vi "VisualizeAppLSE.vi"() -> ()   [LabVIEW 2014, in "Visualization.lvlib" / "VisualizeAppLSE.lvclass"]
uses:
  VisualizeAppLSE.lvclass
  Modules/AppModule/PublicAPI/Arguments/Broadcasts/clStatUpdate.ctl
  VisializeBase_class/Requests/clUserEventType.ctl
  Modules/EventPlugins/EventPluginBaseClass/TypeDefs/clEvtReportArray.ctl
  Modules/EventPlugins/EventPluginBaseClass/TypeDefs/clEvtReport.ctl
  VisualizeAppBase_class.lvclass/VisualizeAppBase_class.ctl
  Modules/AppPlugins/LSEPlugin/PublicAPI/Typedefs/LSEOutput.ctl
  Modules/AppPlugins/LSEPlugin/PublicAPI/Typedefs/LSEConfig.ctl
  VisualizeAppLSE.lvclass/VisualizeAppLSE.ctl
  <vilib>/event_ctls.llb/usereventprio.ctl
  VisualizeAppBase/Accessors/Write clEvtReportArray.vi
  Accessors/Write LSEOutput.vi
  Accessors/Read LSEOutput.vi
  Accessors/Write tve.vi
  Accessors/Write EvtParams.vi
  VisualizeAppBase/Accessors/Read clEvtReportArray.vi
  Accessors/Read tve.vi
  <vilib>/Analysis/BLAS.llb/dnrm2 - Vector 2-Norm (DBL).vi
  <vilib>/Utility/error.llb/Error Cluster From Error Code.vi
  <vilib>/ErrorRing/Error Ring.xnode
  <userlib>/NIST/NISTErrorLib/NISTErrorLib.lvlib
  VisializeBase_class/VisualizeBase_class.lvclass
  Modules/AppModule/AppModule.lvlib
  Modules/EventPlugins/EventPluginBaseClass/EventPluginBaseClass.lvclass
  Modules/PmuImpairModule/PmuImpairModule.lvlib
  Modules/EventModule/EventModule.lvlib
  <vilib>/Analysis/NI_AALBLAS.lvlib
  Modules/AppPlugins/LSEPlugin/LSEPlugin.lvclass
panel:
  out "TVE":waveform(dbl)(graph)
  out "PMU Number":dbl
  in  "Bus Number":u16(ring) items=["1"=1, "2"=2, "3"=3, "4"=4, "5"=5]
  out "IEEE Bus System":u32
  out "% Observed Buses":dbl
  out "Angle estimate":waveform(dbl)[](graph)
  out "Magnitude estimate":waveform(dbl)[](graph)
  out "Event Parameters":dbl[][](array[numeric])
  in  "btnStop":bool
  out "Status Broadcasts":string
  in  "QueName":string="VisAppQue"
  out "TSE":waveform(dbl)[](graph)
  in  "restart VI":bool
  out "Error Array":errorcluster[][](array[cluster])
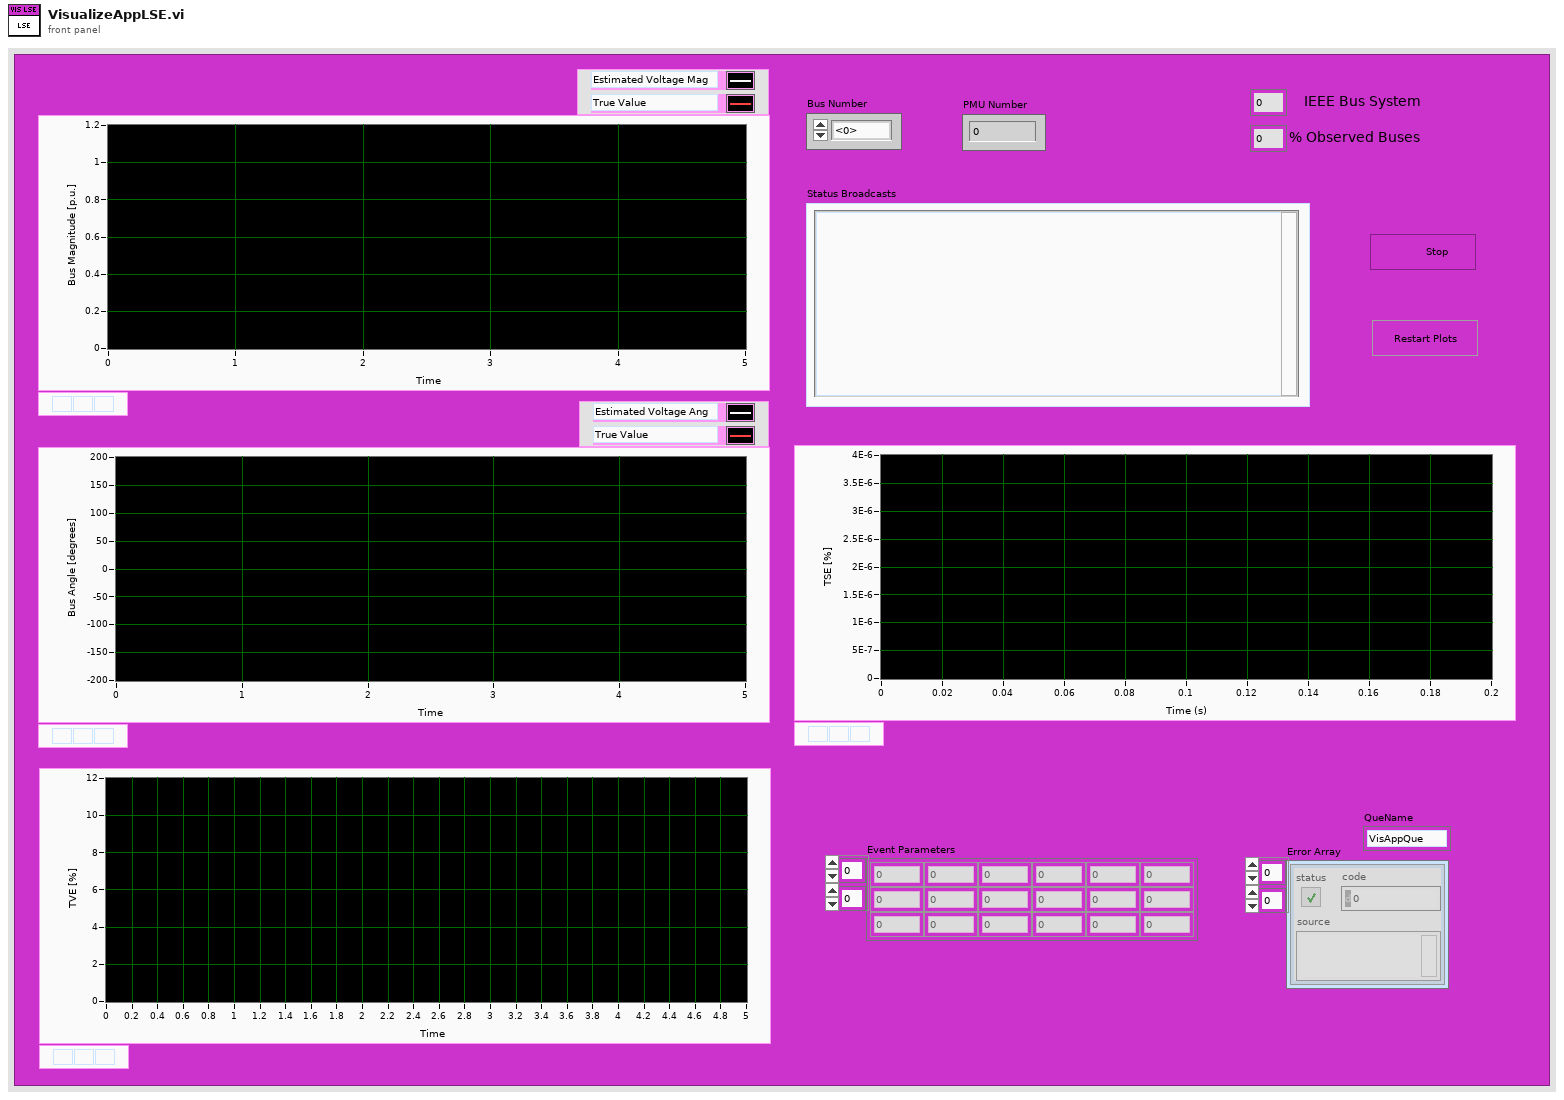
[diagram p1: front panel]
types:
  T1 = typedef "EventPlugins.lvlib/EventPluginBaseClass.lvclass/clEvtReportArray.ctl" = T2[]
  T2 = typedef "EventPlugins.lvlib/EventPluginBaseClass.lvclass/clEvtReport.ctl" = cluster{"Timestamp":dbl, "Synx":cdb[], "Freq":dbl, "ROCOF":dbl, "ID":i16}
  T3 = typedef "AppPlugins.lvlib/LSEPlugin.lvclass/LSEOutput.ctl" = cluster{"SystemVoltagesRef":cdb[][], "Vestimate":cdb[][], "LSEConfig":T4, "Bus":dbl[]}
  T4 = typedef "AppPlugins.lvlib/LSEPlugin.lvclass/LSEConfig.ctl" = cluster{"NoiseVariance":dbl, "IEEESystem":u32, "PMULocations":u32[], "Vindex":i32, "Iindex":i32, "DynamicRef":string}
  T5 = typedef "Visualization.lvlib/VisualizeBase_class.lvclass/clUserEventType.ctl" = cluster{"BusIndex":i8, "Data":variant}
  T6 = typedef "usereventprio.ctl" = enum32{"high priority", "normal priority"}
  T7 = typedef "AppModule.lvlib/clStatUpdate.ctl" = cluster{"Status":string}
  T8 = typedef "Visualization.lvlib/VisualizeBase_class.lvclass/clRequestEvents.ctl" = cluster{"StopRequest":refnum<user-event>}
  T9 = typedef "AppModule.lvlib/clBroadcastEvents.ctl" = cluster{"DidInit":refnum<user-event>, "StatusUpdate":refnum<user-event>, "ErrorReport":refnum<user-event>, "DidStop":refnum<user-event>, "PathToINI":refnum<user-event>, "InputData":refnum<user-event>, "OutputData":refnum<user-event>, "BcAppInfo":refnum<user-event>, "ConfigData":refnum<user-event>}
  T10 = typedef "PmuImpairModule.lvlib/clBroadcastEvents.ctl" = cluster{"DidInit":refnum<user-event>, "StatusUpdate":refnum<user-event>, "ErrorReport":refnum<user-event>, "DidStop":refnum<user-event>, "ImpairConfig":refnum<user-event>, "ImpairParams":refnum<user-event>, "ImpairReports":refnum<user-event>, "PathToPlugin":refnum<user-event>, "BusNumber":refnum<user-event>}
  T11 = typedef "EventModule.lvlib/clBroadcastEvents.ctl" = cluster{"DidInit":refnum<user-event>, "StatusUpdate":refnum<user-event>, "ErrorReport":refnum<user-event>, "DidStop":refnum<user-event>, "ReadEvtConfig":refnum<user-event>, "ReadTimeArray":refnum<user-event>, "ReadEvtParams":refnum<user-event>, "GetEvtReportArray":refnum<user-event>, "ReadPathToPlugin":refnum<user-event>, "GetEvtSignal":refnum<user-event>, "ReadBusNumber":refnum<user-event>}
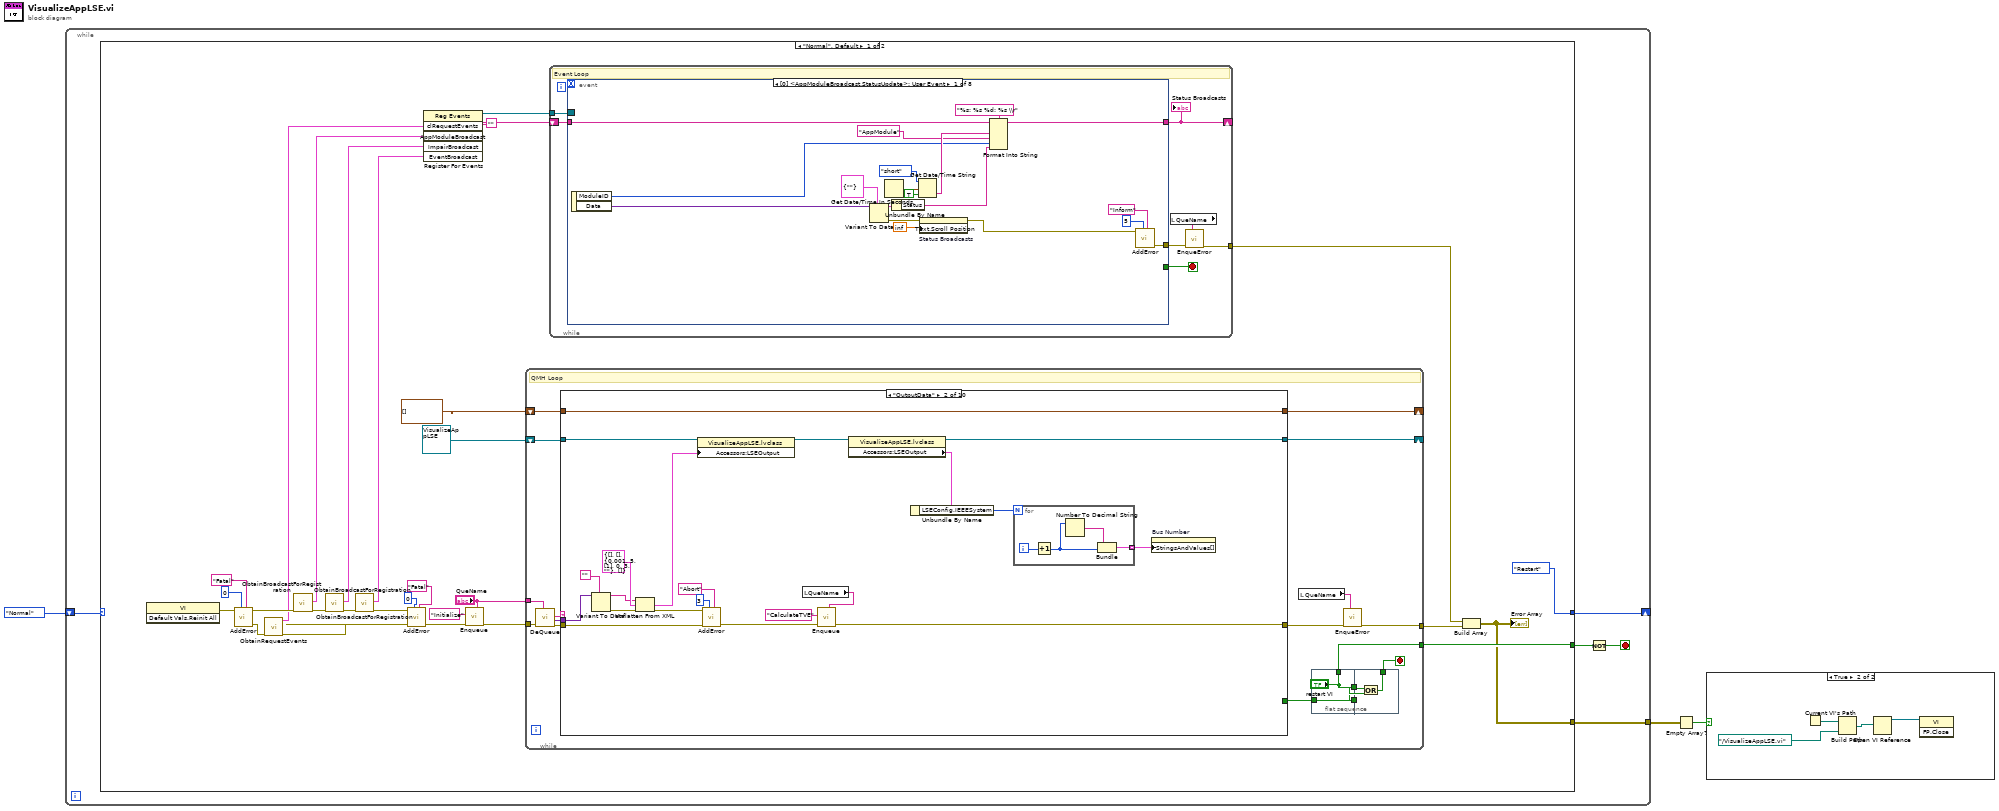
[diagram p0: block diagram]
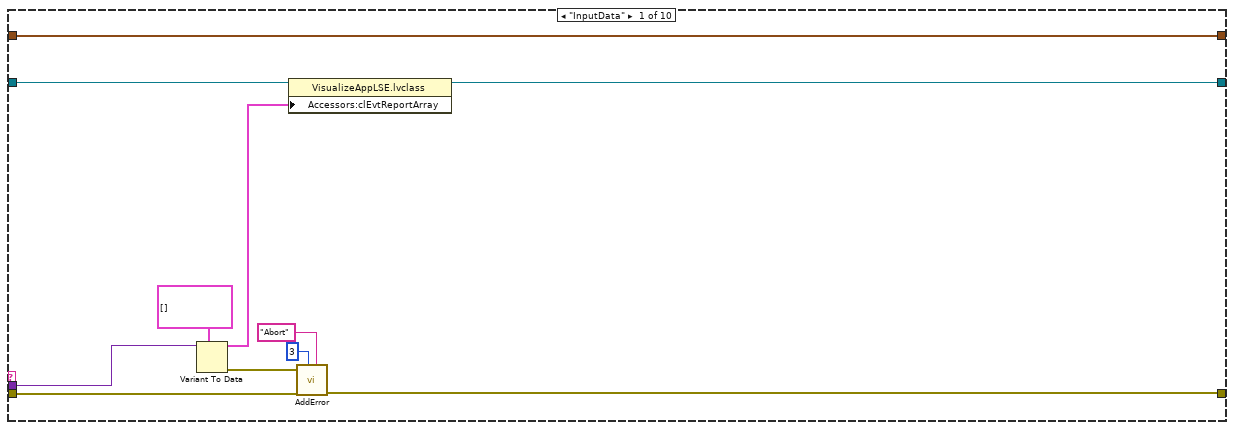
[diagram p3: hidden frame]
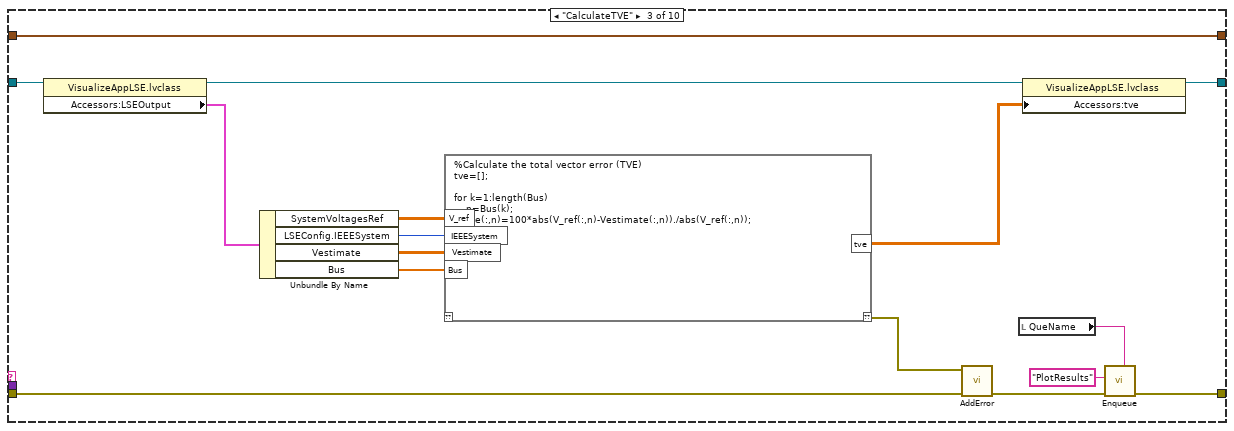
[diagram p4: hidden frame]
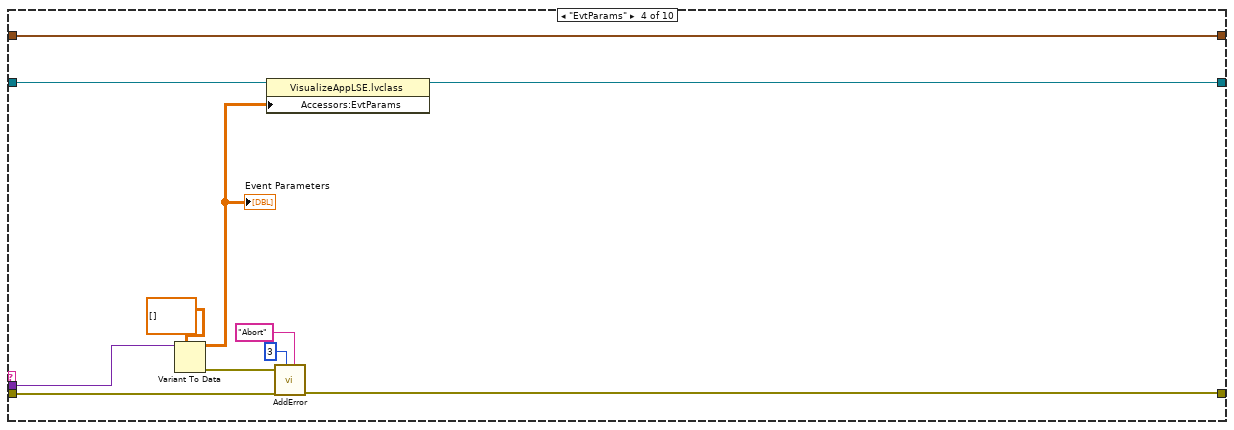
[diagram p5: hidden frame]
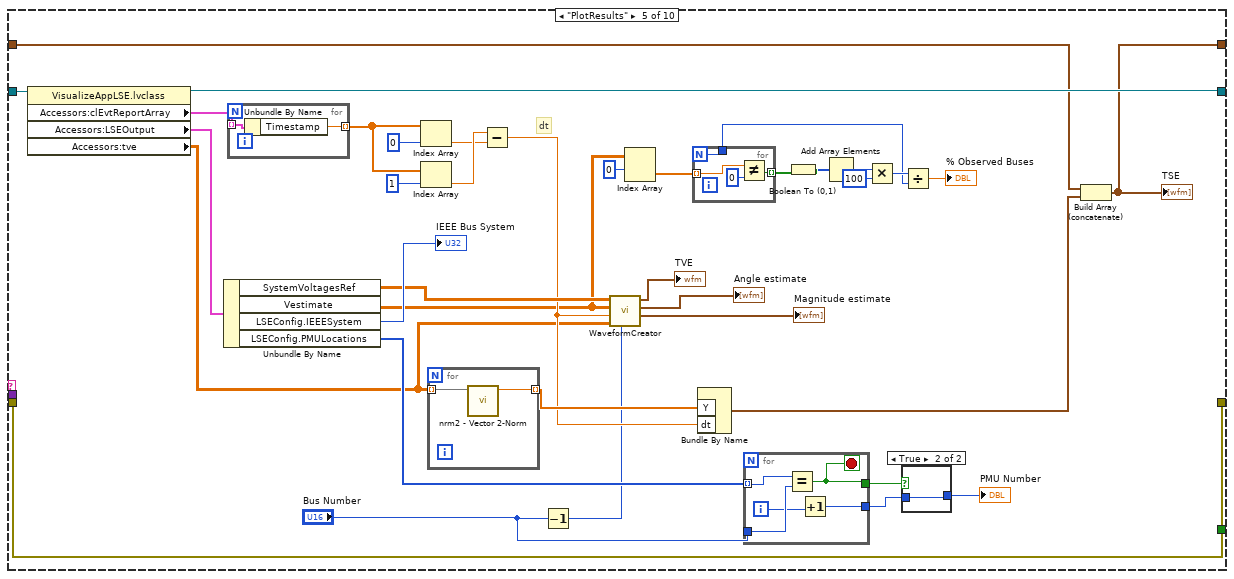
[diagram p6: hidden frame]
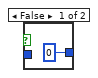
[diagram p7: hidden frame]
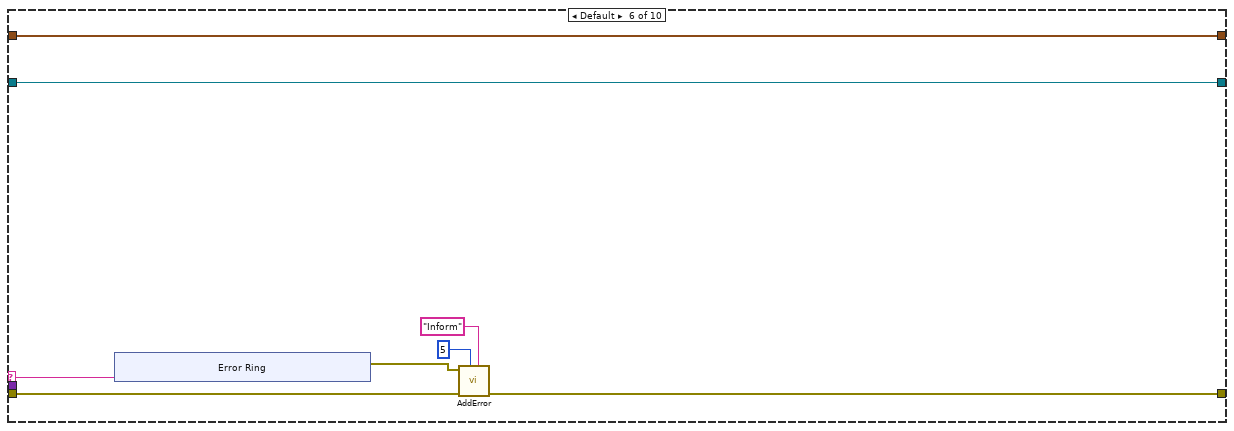
[diagram p8: hidden frame]
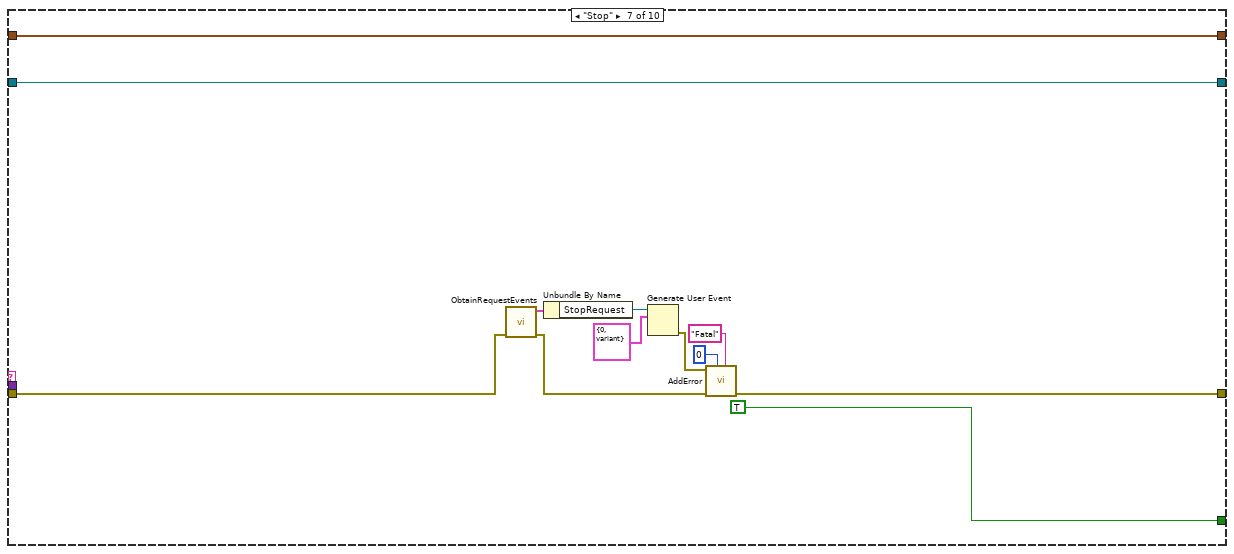
[diagram p9: hidden frame]
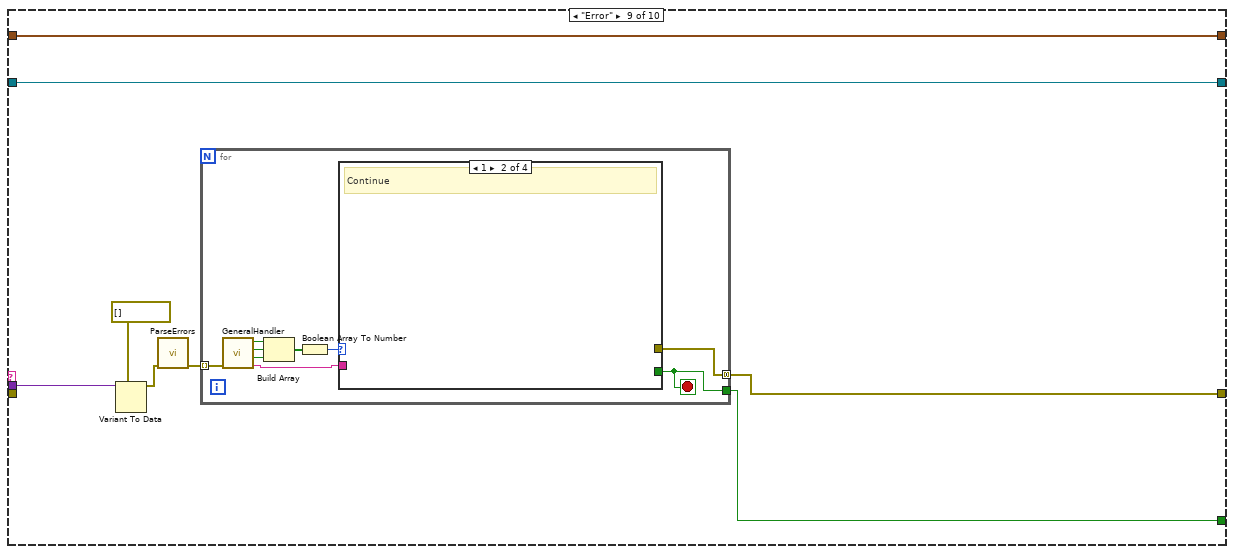
[diagram p11: hidden frame]
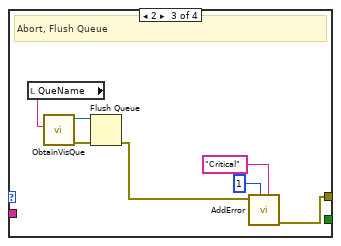
[diagram p13: hidden frame]
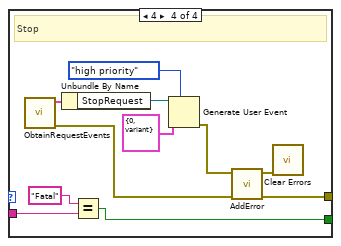
[diagram p14: hidden frame]
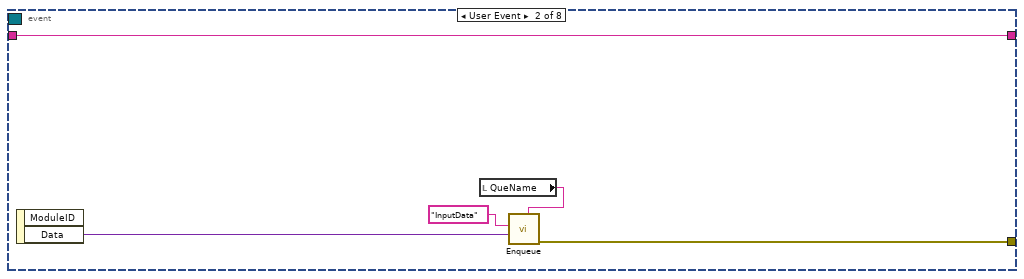
[diagram p16: hidden frame]
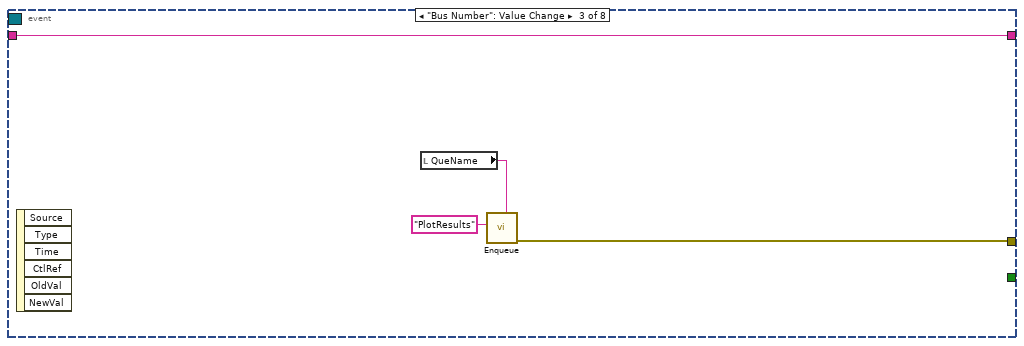
[diagram p17: hidden frame]
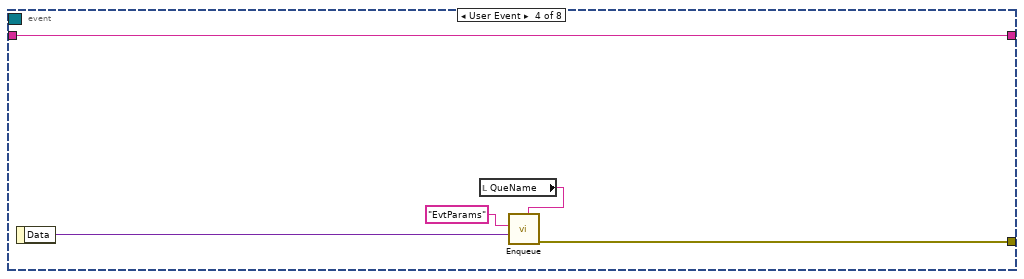
[diagram p18: hidden frame]
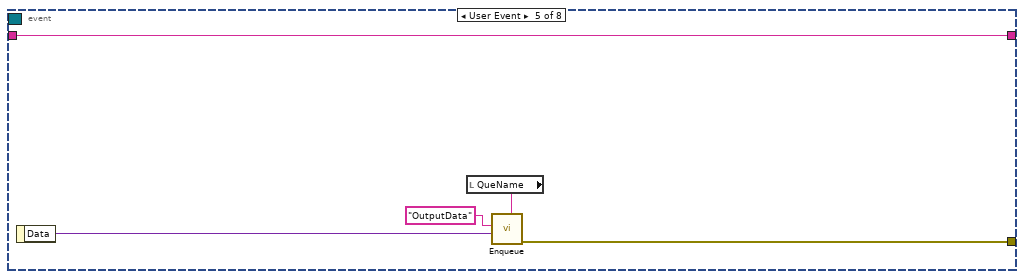
[diagram p19: hidden frame]
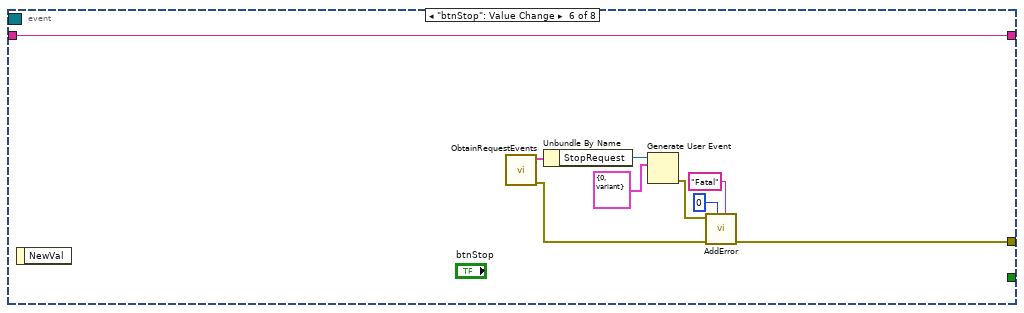
[diagram p20: hidden frame]
diagram:
  n1 = while {
    shift-right: [w5] -> _
    shift-left: enum16{"Normal", "Restart"}."Normal" -> [w6]
    tunnel: [w4] -> w1
    stop <- w7 stop-if-true
    n2 = case shown="\"Normal\", Default" w6 {
      tunnel: [w13 TRUE] -> w8
      tunnel: [enum16{"Normal", "Restart"}."Restart" enum16{"Normal", "Restart"}."Normal"] -> w5
      tunnel: [w10 errorcluster[][] []] -> w4
      frame "Normal", Default {
        n3 = invoke class="VI" method="Default Vals.Reinit All"() -> (error out=w19:errorcluster)  [unwired: 3 in, 2 out]
        n4 = call <userlib>:"AddError.vi"("Severity"="Fatal", "Priority"=u8 0, "error in (no error)"=w19) -> ("ErrorArray"=w34:errorcluster[], "error out"=w33:errorcluster)  [unwired: 7 in]
        n5 = call "ObtainRequestEvents.vi"("Error"=w34) -> ("Error"=w30:errorcluster[], "clRequestEvents"=w32:T8)  [unwired: 9 in]
        n6 = call "ObtainBroadcastForRegistration.vi"("error in (no error)"=w33) -> ("error out"=w18:errorcluster, "AppModuleBroadcast"=w31:T9)  [unwired: 9 in]
        n7 = call "ObtainBroadcastForRegistration.vi"("error in (no error)"=w18) -> ("error out"=w17:errorcluster, "ImpairBroadcast"=w16:T10)  [unwired: 9 in]
        n8 = call "ObtainBroadcastForRegistration.vi"("error in (no error)"=w17) -> ("error out"=w15:errorcluster, "EventBroadcast"=w14:T11)  [unwired: 9 in]
        n9 = call <userlib>:"AddError.vi"("Severity"="Fatal", "Priority"=u8 0, "ErrorArray"=w30, "error in (no error)"=w15) -> ("ErrorArray"=w28:errorcluster[])  [unwired: 6 in, 1 out]
        n10 = register-events(w32, w31, w16, w14) -> (reference out=w23:refnum<event-registration>)  [unwired: 2 in, 1 out]
        n11 = call "Enqueue.vi"("QueName"="QueName", "Error"=w28, "Message"="Initialize") -> ("Error"=w25:errorcluster[])  [unwired: 8 in]
        n12 = while {
          tunnel: w25 -> [w53]
          tunnel: "QueName" -> [w52]
          tunnel: [w46] -> w22
          shift-right: [w44] -> _
          shift-left: refnum<class "VisualizeAppLSE.lvclass"> refnum ("Visualization.lvlib:VisualizeAppLSE.lvclass") -> [w45]
          shift-right: [w42] -> _
          shift-left: waveform(dbl)[] [] -> [w43]
          tunnel: [w41] -> w13
          stop <- w37 stop-if-true
          # "QMH Loop"
          n13 = call "DeQueue.vi"("QueName"=w52, "Error"=w53) -> ("Error"=w49:errorcluster[], "Data"=w50:variant, "Message"=w51:string)  [unwired: 7 in]
          n14 = case shown="\"OutputData\"" w51 {
            selector: w51 -> [_ _ _ _ _ w181 _ _ _ _]
            tunnel: w50 -> [w67 w89 _ w119 _ _ _ _ w208 _]
            tunnel: w49 -> [w63 w88 w99 w116 w124 w180 w192 w203 _ w239]
            tunnel: [w62 w84 w108 w115 w124 w176 w193 w203 w210 w239] -> w48
            tunnel: [_ _ _ _ _ _ TRUE _ w211 _] -> w39
            tunnel: w45 -> [w69 w90 w106 w121 w158 w175 w190 w202 w205 w240]
            tunnel: [w68 w79 w104 w120 w157 w175 w190 w202 w205 w240] -> w44
            tunnel: w43 -> [w59 w81 w107 w111 w155 w174 w189 w201 w204 w241]
            tunnel: [w59 w81 w107 w111 w146 w174 w189 w201 w204 w241] -> w42
            frame "InputData" {
              n15 = Variant To Data(type=T1 [] ("clEvtReportArray"), Variant=w67) -> (data=w65:T1, error out=w64:errorcluster)  [unwired: 1 in]
              n16 = property class="VisualizeAppLSE.lvclass"(reference=w69, "Accessors:clEvtReportArray"=w65) -> (reference out=w68:refnum<class "VisualizeAppLSE.lvclass">)  [unwired: 1 in, 1 out]
              n17 = call <userlib>:"AddError.vi"("Severity"="Abort", "Priority"=u8 3, "ErrorArray"=w63, "error in (no error)"=w64) -> ("ErrorArray"=w62:errorcluster[])  [unwired: 6 in, 1 out]
            }
            frame "OutputData" {
              n18 = Variant To Data(type="", Variant=w89) -> (data=w73:string, error out=w72:errorcluster)  [unwired: 1 in]
              n19 = Unflatten From XML(xml string=w73, type=T3 {"SystemVoltagesRef"=[], "Vestimate"=[], "LSEConfig"={"NoiseVariance"=0.001, "IEEESystem"=5, "PMULocations"=[1], "Vindex"=0, "Iindex"=3, "DynamicRef"=""}, "Bus"=[]} ("LSEOutput"), error in (no error)=w72) -> (value=w70:T3, error out=w71:errorcluster)
              n20 = property class="VisualizeAppLSE.lvclass"(reference=w90, "Accessors:LSEOutput"=w70) -> (reference out=w80:refnum<class "VisualizeAppLSE.lvclass">)  [unwired: 1 in, 1 out]
              n21 = call <userlib>:"AddError.vi"("Severity"="Abort", "Priority"=u8 3, "ErrorArray"=w88, "error in (no error)"=w71) -> ("ErrorArray"=w85:errorcluster[])  [unwired: 6 in, 1 out]
              n22 = local read "QueName"() -> (w82:string)
              n23 = call "Enqueue.vi"("QueName"=w82, "Error"=w85, "Message"="CalculateTVE") -> ("Error"=w84:errorcluster[])  [unwired: 8 in]
              n24 = property class="VisualizeAppLSE.lvclass"(reference=w80) -> (reference out=w79:refnum<class "VisualizeAppLSE.lvclass">, "Accessors:LSEOutput"=w78:T3)  [unwired: 1 in, 1 out]
              n25 = Unbundle By Name(w78) -> ("LSEConfig.IEEESystem"=w77:u32)
              n26 = for {
                N: w77 -> [_]
                tunnel: [w93] -> w76 mode=indexing
                i -> [w92]
                n27 = Increment(x=w92) -> (x+1=w91:i32)
                n28 = Number To Decimal String(number=w91) -> (decimal integer string=w94:string)  [unwired: 1 in]
                n29 = Bundle(w94, w91) -> (w93:cluster{string, i32})  [unwired: 1 in]
              }
              n30 = property on="Bus Number" class="Ring (strict)"("StringsAndValues[]"=w76) -> ()  [unwired: 2 in, 2 out]
            }
            frame "CalculateTVE" {
              n31 = property class="VisualizeAppLSE.lvclass"(reference=w106) -> (reference out=w105:refnum<class "VisualizeAppLSE.lvclass">, "Accessors:LSEOutput"=w97:T3)  [unwired: 1 in, 1 out]
              n32 = Unbundle By Name(w97) -> ("SystemVoltagesRef"=w95:cdb[][], "LSEConfig.IEEESystem"=w103:u32, "Vestimate"=w102:cdb[][], "Bus"=w101:dbl[])
              n33 = script code="%Calculate the total vector error (TVE)\ntve=[];\n\nfor k=1:length(Bus)\n    n=Bus(k);\n    tve(:,n)=100*abs(V_ref(:,n)-Vestimate(:,n))./abs(V_ref(:,n));  \nend"("V_ref"=w95, "IEEESystem"=w103, "Vestimate"=w102, "Bus"=w101) -> ("??"=w100:errorcluster, "tve"=w96:dbl[][])  [unwired: 1 in]
              n34 = call <userlib>:"AddError.vi"("ErrorArray"=w99, "error in (no error)"=w100) -> ("ErrorArray"=w98:errorcluster[])  [unwired: 8 in, 1 out]
              n35 = local read "QueName"() -> (w109:string)
              n36 = property class="VisualizeAppLSE.lvclass"(reference=w105, "Accessors:tve"=w96) -> (reference out=w104:refnum<class "VisualizeAppLSE.lvclass">)  [unwired: 1 in, 1 out]
              n37 = call "Enqueue.vi"("QueName"=w109, "Error"=w98, "Message"="PlotResults") -> ("Error"=w108:errorcluster[])  [unwired: 8 in]
            }
            frame "EvtParams" {
              n38 = Variant To Data(type=dbl[][] [], Variant=w119) -> (data=w118:dbl[][], error out=w117:errorcluster)  [unwired: 1 in]
              "Event Parameters" <- w118
              n39 = property class="VisualizeAppLSE.lvclass"(reference=w121, "Accessors:EvtParams"=w118) -> (reference out=w120:refnum<class "VisualizeAppLSE.lvclass">)  [unwired: 1 in, 1 out]
              n40 = call <userlib>:"AddError.vi"("Severity"="Abort", "Priority"=u8 3, "ErrorArray"=w116, "error in (no error)"=w117) -> ("ErrorArray"=w115:errorcluster[])  [unwired: 6 in, 1 out]
            }
            frame "PlotResults" {
              # "dt"
              n41 = property class="VisualizeAppLSE.lvclass"(reference=w158) -> (reference out=w157:refnum<class "VisualizeAppLSE.lvclass">, "Accessors:clEvtReportArray"=w153:T1, "Accessors:LSEOutput"=w152:T3, "Accessors:tve"=w122:dbl[][])  [unwired: 1 in, 1 out]
              n42 = Unbundle By Name(w152) -> ("SystemVoltagesRef"=w131:cdb[][], "Vestimate"=w128:cdb[][], "LSEConfig.IEEESystem"=→"IEEE Bus System":u32, "LSEConfig.PMULocations"=w127:u32[])
              n43 = for {
                tunnel: w153 -> [w173] mode=indexing
                tunnel: [w172] -> w149 mode=indexing
                n44 = Unbundle By Name(w173) -> ("Timestamp"=w172:dbl)
              }
              n45 = Index Array(array=w149, index=0) -> (element=w147:dbl)
              n46 = Index Array(array=w149, index=1) -> (element=w148:dbl)
              n47 = for {
                tunnel: [w170] -> w151 mode=indexing
                tunnel: w122 -> [w171] mode=indexing
                n48 = call-poly <vilib>:"nrm2 - Vector 2-Norm.vi"("x"=w171) -> ("dnrm2"=w170:dbl)  [unwired: 9 in, 1 out]
              }
              n49 = Subtract(x=w148, y=w147) -> (x-y=w130:dbl)
              n50 = Decrement(x="Bus Number") -> (x-1=w123:u16)
              n51 = call "WaveformCreator.vi"("BusNumber"=w123, "error"=w122, "dt"=w130, "Vestimate"=w128, "SystemVoltagesRef"=w131) -> ("MagnitudeEstimate"=→"Magnitude estimate":waveform(dbl)[], "AngleEstimate"=→"Angle estimate":waveform(dbl)[], "TVE"=→"TVE":waveform(dbl))  [unwired: 4 in]
              n52 = Index Array(array=w128, index (row)=0) -> (element=w144:cdb[])  [unwired: 1 in]
              n53 = for {
                N -> [w168]
                tunnel: w144 -> [w166] mode=indexing
                tunnel: [w169] -> w143 mode=indexing
                tunnel: [w168] -> w138
                n54 = Not Equal?(x=w166, y=0) -> (x != y?=w169:bool)
              }
              n55 = Bundle By Name("Y"=w151, "dt"=w130) -> (w156:waveform(dbl))  [unwired: 1 in]
              n56 = for {
                tunnel: w127 -> [w163] mode=indexing
                tunnel: "Bus Number" -> [w162]
                tunnel: [w160] -> w133
                tunnel: [w159] -> w134
                i -> [w161]
                stop <- w159 stop-if-true
                n57 = Equal?(x=w163, y=w162) -> (x = y?=w159:bool)
                n58 = Increment(x=w161) -> (x+1=w160:i32)
              }
              n59 = Boolean To (0,1)(Boolean=w143) -> (0, 1=w142:i16[])
              n60 = Add Array Elements(numeric array=w142) -> (sum=w141:i16)
              n61 = Multiply(x=w141, y=i16 100) -> (x*y=w139:i16)
              n62 = case shown="True" w134 {
                tunnel: [0 w165] -> w132
                tunnel: w133 -> [_ w165]
                frame False {
                }
                frame True {
                }
              }
              "PMU Number" <- w132
              n63 = Divide(x=w139, y=w138) -> (x/y=→"% Observed Buses":dbl)
              n64 = Build Array (concatenate)(w155, w156) -> (w146:waveform(dbl)[])
              "TSE" <- w146
            }
            frame Default {
              n65 = xnode "Error Ring"("parameter 0"=w181) -> ("error out"=w179:errorcluster)
              n66 = call <userlib>:"AddError.vi"("Severity"="Inform", "Priority"=u8 5, "ErrorArray"=w180, "error in (no error)"=w179) -> ("ErrorArray"=w176:errorcluster[])  [unwired: 6 in, 1 out]
            }
            frame "Stop" {
              n67 = call "ObtainRequestEvents.vi"("Error"=w192) -> ("Error"=w191:errorcluster[], "clRequestEvents"=w194:T8)  [unwired: 9 in]
              n68 = Unbundle By Name(w194) -> ("StopRequest"=w195:refnum<user-event>)
              n69 = Generate User Event(user event=w195, event data cluster=T5 {"BusIndex"=0, "Data"=variant} ("clEventType")) -> (error out=w197:errorcluster)  [unwired: 2 in, 1 out]
              n70 = call <userlib>:"AddError.vi"("Severity"="Fatal", "Priority"=u8 0, "ErrorArray"=w191, "error in (no error)"=w197) -> ("ErrorArray"=w193:errorcluster[])  [unwired: 6 in, 1 out]
            }
            frame "Initialize" {
            }
            frame "Error" {
              n71 = Variant To Data(type=errorcluster[] [], Variant=w208) -> (data=w206:errorcluster[])  [unwired: 1 in, 1 out]
              n72 = call <userlib>:"ParseErrors.vi"("ErrorArray"=w206) -> ("ErrorArray"=w209:errorcluster[])  [unwired: 8 in, 2 out]
              n73 = for {
                tunnel: w209 -> [w220] mode=indexing
                tunnel: [w214] -> w210 mode=concatenating
                tunnel: [w212] -> w211
                stop <- w212 stop-if-true
                n74 = call <userlib>:"GeneralHandler.vi"("error in (no error)"=w220) -> ("Severity"=w213:string, "Stop"=w217:bool, "Abort"=w218:bool, "Continue"=w219:bool)  [unwired: 7 in]
                n75 = Build Array(w219, w218, w217) -> (w216:bool[])
                n76 = Boolean Array To Number(Boolean array=w216) -> (number=w215:u32)
                n77 = case shown="1" w215 {
                  tunnel: [_ _ w225 w236] -> w214
                  tunnel: w213 -> [_ _ _ w230]
                  tunnel: [_ _ _ w228] -> w212
                  frame 0, Default {
                    # "No Dialog"
                  }
                  frame 1 {
                    # "Continue"
                  }
                  frame 2 {
                    # "Abort, Flush Queue"
                    n78 = local read "QueName"() -> (w221:string)
                    n79 = call "ObtainVisQue.vi"("QueName"=w221) -> ("error out"=w227:errorcluster, "queue out"=w226:refnum<queue>)  [unwired: 9 in]
                    n80 = Flush Queue(queue=w226, error in (no error)=w227) -> (error out=w224:errorcluster)  [unwired: 2 out]
                    n81 = call <userlib>:"AddError.vi"("Severity"="Critical" ("String"), "Priority"=u8 1, "error in (no error)"=w224) -> ("ErrorArray"=w225:errorcluster[])  [unwired: 7 in, 1 out]
                  }
                  frame 4 {
                    # "Stop"
                    n82 = call "ObtainRequestEvents.vi"() -> ("Error"=w234:errorcluster[], "clRequestEvents"=w238:T8)  [unwired: 10 in]
                    n83 = Unbundle By Name(w238) -> ("StopRequest"=w237:refnum<user-event>)
                    n84 = Equal?(x="Fatal", y=w230) -> (x = y?=w228:bool)
                    n85 = Generate User Event(priority (normal)=usereventprio."high priority", user event=w237, event data cluster=T5 {"BusIndex"=0, "Data"=variant} ("event data")) -> (error out=w235:errorcluster)  [unwired: 1 in, 1 out]
                    n86 = call <userlib>:"AddError.vi"("ErrorArray"=w234, "error in (no error)"=w235) -> ("ErrorArray"=w236:errorcluster[], "error out"=w231:errorcluster)  [unwired: 8 in]
                    n87 = call <vilib>:"Clear Errors.vi"("error in (no error)"=w231) -> ()  [unwired: 5 in, 2 out]
                  }
                }
              }
            }
            frame "Restart" {
            }
          }
          n88 = local read "QueName"() -> (w47:string)
          n89 = flat-sequence {
            tunnel: ["restart VI"] -> w41
            tunnel: ["restart VI"] -> w40
            tunnel: w39 -> [w54]
            tunnel: [w54] -> w38
            tunnel: w40 -> [w58]
            tunnel: w38 -> [w57]
            tunnel: [w56] -> w37
            frame #0 {
            }
            frame #1 {
              n90 = Or(x=w57, y=w58) -> (x .or. y?=w56:bool)
            }
          }
          n91 = call "EnqueError.vi"("QueName"=w47, "Error"=w48) -> ("Error"=w46:errorcluster[])  [unwired: 9 in]
        }
        n92 = while {
          tunnel: [w247] -> w21
          tunnel: w23 -> [w245]
          shift-right: [w242] -> _
          shift-left: "" -> [w243]
          stop <- w244 stop-if-true
          # "Event Loop"
          n93 = event shown="[0] <AppModuleBroadcast.StatusUpdate>: User Event" {
            selector: w245 -> [_ _ _ _ _ _ _ _]
            dyn-events: _ -> [_ _ _ _ _ _ _ _]
            timeout: _ -> [_ _ _ _ _ _ _ _]
            tunnel: [w256 w271 w273 w280 w285 w290 w298 w302] -> w248
            tunnel: [_ _ _ _ _ _ TRUE TRUE] -> w244
            tunnel: w243 -> [w267 w269 w276 w278 w282 w287 w296 w307]
            tunnel: [w260 w269 w276 w278 w282 w287 w296 w307] -> w242
            event User Event {
              n94 = event-data() -> ("ModuleID"=w250:i32, "Data"=w266:variant)  [unwired: 1 in]
              n95 = Variant To Data(type=T7 {"Status"=""} ("clStatUpdate"), Variant=w266) -> (data=w264:T7, error out=w257:errorcluster)  [unwired: 1 in]
              n96 = Get Date/Time In Seconds() -> (seconds since 1Jan1904=w261:timestamp)
              n97 = Unbundle By Name(w264) -> ("Status"=w251:string)
              n98 = Get Date/Time String(date format (0)=enum16{"short", "long", "abbreviated"}."short", seconds (now)=w261, want seconds? (F)=TRUE) -> (time string=w258:string)  [unwired: 1 out]
              n99 = property on="Status Broadcasts" class="Str"(error in=w257, "Text.Scroll Position"=inf) -> (error out=w255:errorcluster)  [unwired: 1 in, 1 out]
              n100 = Format Into String(format string="%s: %s %d: %s \\r", initial string=w267, w258, "AppModule", w250, w251) -> (resulting string=w260:string)  [unwired: 1 in, 1 out]
              n101 = call <userlib>:"AddError.vi"("Severity"="Inform", "Priority"=u8 5, "error in (no error)"=w255) -> ("ErrorArray"=w256:errorcluster[])  [unwired: 7 in, 1 out]
            }
            event User Event {
              n102 = event-data() -> ("Data"=w272:variant)  [unwired: 1 in, 1 out]
              n103 = local read "QueName"() -> (w268:string)
              n104 = call "Enqueue.vi"("QueName"=w268, "Data"=w272, "Message"="InputData") -> ("Error"=w271:errorcluster[])  [unwired: 8 in]
            }
            event "Bus Number": Value Change {
              n105 = event-data() -> ()  [unwired: 1 in, 6 out]
              n106 = local read "QueName"() -> (w275:string)
              n107 = call "Enqueue.vi"("QueName"=w275, "Message"="PlotResults") -> ("Error"=w273:errorcluster[])  [unwired: 9 in]
            }
            event User Event {
              n108 = event-data() -> ("Data"=w281:variant)  [unwired: 1 in]
              n109 = local read "QueName"() -> (w277:string)
              n110 = call "Enqueue.vi"("QueName"=w277, "Data"=w281, "Message"="EvtParams") -> ("Error"=w280:errorcluster[])  [unwired: 8 in]
            }
            event User Event {
              n111 = event-data() -> ("Data"=w286:variant)  [unwired: 1 in]
              n112 = local read "QueName"() -> (w283:string)
              n113 = call "Enqueue.vi"("QueName"=w283, "Data"=w286, "Message"="OutputData") -> ("Error"=w285:errorcluster[])  [unwired: 8 in]
            }
            event "btnStop": Value Change {
              n114 = event-data() -> ()  [unwired: 1 in, 1 out]
              n115 = call "ObtainRequestEvents.vi"() -> ("Error"=w292:errorcluster[], "clRequestEvents"=w295:T8)  [unwired: 10 in]
              n116 = Unbundle By Name(w295) -> ("StopRequest"=w294:refnum<user-event>)
              n117 = Generate User Event(user event=w294, event data cluster=T5 {"BusIndex"=0, "Data"=variant} ("clEventType")) -> (error out=w291:errorcluster)  [unwired: 2 in, 1 out]
              n118 = call <userlib>:"AddError.vi"("Severity"="Fatal", "Priority"=u8 0, "ErrorArray"=w292, "error in (no error)"=w291) -> ("ErrorArray"=w290:errorcluster[])  [unwired: 6 in, 1 out]
            }
            event User Event {
              n119 = event-data() -> ()  [unwired: 1 in, 1 out]
              n120 = local read "QueName"() -> (w300:string)
              n121 = call "Enqueue.vi"("QueName"=w300, "Priority? (F)"=TRUE, "Message"="Stop") -> ("Error"=w298:errorcluster[])  [unwired: 8 in]
            }
            event "restart VI": Value Change {
              n122 = event-data() -> ()  [unwired: 1 in, 5 out]
              n123 = local read "QueName"() -> (w304:string)
              n124 = call "Enqueue.vi"("QueName"=w304, "Priority? (F)"=TRUE, "Message"="Restart") -> ("Error"=w302:errorcluster[])  [unwired: 8 in]
            }
          }
          "Status Broadcasts" <- w242
          n125 = local read "QueName"() -> (w246:string)
          n126 = call "EnqueError.vi"("QueName"=w246, "Error"=w248) -> ("Error"=w247:errorcluster[])  [unwired: 9 in]
        }
        n127 = Build Array(w21, w22) -> (w10:errorcluster[][])
        "Error Array" <- w10
      }
      frame "Restart" {
        # "Calls the VI server reintializing the VI"
        n128 = control-ref of="This VI"() -> (w309:refnum<vi>)
        n129 = invoke class="VI" method="Default Vals.Reinit All"(reference=w309) -> ()  [unwired: 2 in, 3 out]
      }
    }
    n130 = Not(x=w8) -> (.not. x?=w7:bool)
  }
  n131 = Empty Array?(array=w1) -> (empty?=w2:bool)
  n132 = case shown="True" w2 {
    frame False {
    }
    frame True {
      n133 = Current VI's Path() -> (path=w314:path)
      n134 = Build Path(base path=w314, name or relative path=path "../VisualizeAppLSE.vi") -> (appended path=w312:path)
      n135 = Open VI Reference(vi path=w312) -> (vi reference=w315:refnum<vi>)  [unwired: 5 in, 1 out]
      n136 = invoke class="VI" method="FP.Close"(reference=w315) -> ()  [unwired: 2 in, 3 out]
    }
  }
